vi "ChannelType_1D-Array-2DPoint-I32.vi"(9 "error in":errorcluster, 11 "Array in":T1[](array[typedef])) -> (1 "error out":errorcluster, 2 "ChannelType":i32, 3 "Array out":T1[](array[typedef]))   [LabVIEW 2020, in "OpenLvVision_OpenCv.lvlib"]
uses:
  TypeDef/Point/2D_PointI32.ctl
  OpenLvVision_OpenCv.lvlib
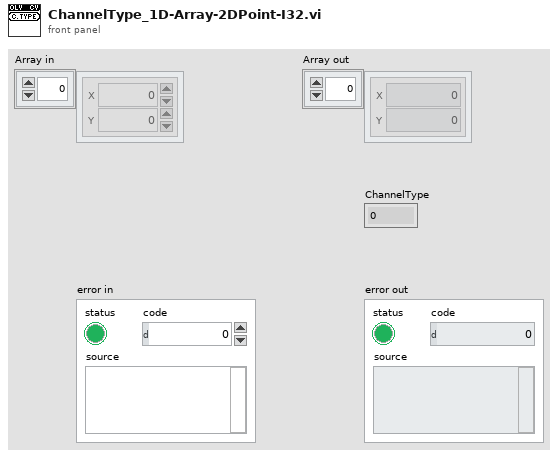
[diagram p1: front panel]
types:
  T1 = typedef "OpenLvVision_OpenCv.lvlib/2D_PointI32.ctl" = cluster{"X":i32, "Y":i32}
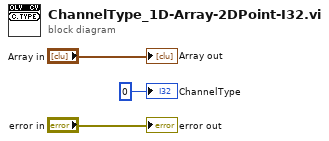
[diagram p0: block diagram]
diagram:
  "error out" <- "error in"
  "Array out" <- "Array in"
  "ChannelType" <- 0
